vi "plot&save.vi"() -> ()   [LabVIEW 2019]
uses:
  <vilib>/Instr/_visa.llb/VISA Configure Serial Port (Instr).vi
panel:
  in  "Choose the data.txt file in the folder":path
  out "Muscle Activity":i32(graph)
  in  "?":bool
  in  "Conect your Arduino and choose the COM port":refnum<visa-resource-name>
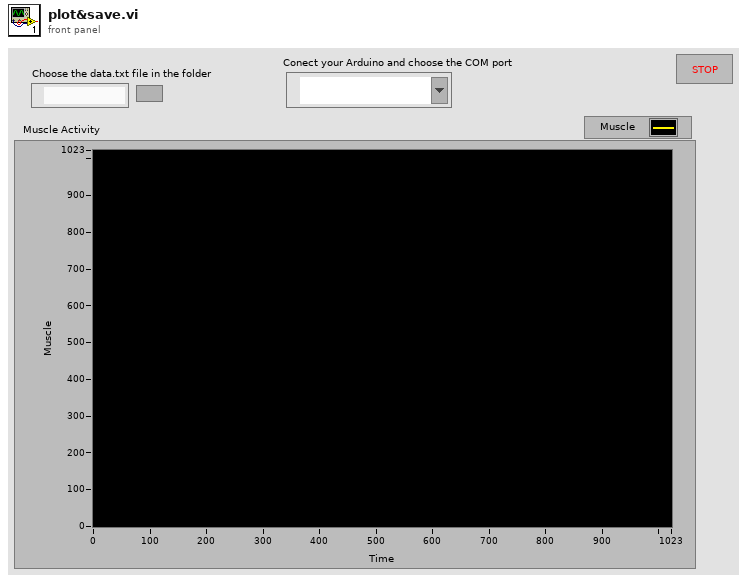
[diagram p1: front panel]
types:
  T1 = enum16{"open", "replace", "create", "open or create", "replace or create", "replace or create with confirmation"}
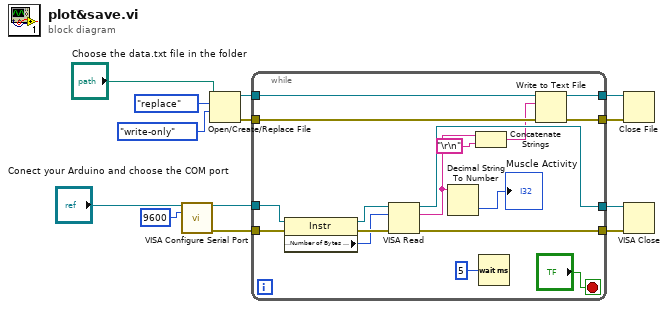
[diagram p0: block diagram]
diagram:
  n1 = call-poly "VISA Configure Serial Port"("VISA resource name"="Conect your Arduino and choose the COM port", "baud rate (9600)"=u32 9600) -> ("VISA resource name out"=w11:refnum<visa-resource-name>, "error out"=w10:errorcluster)  [unwired: 12 in]
  n2 = Open/Create/Replace File(file path (use dialog)="Choose the data.txt file in the folder", operation (0:open)=T1."replace", access (0:read/write)=enum16{"read/write", "read-only", "write-only"}."write-only") -> (refnum out=w7:refnum<file>, error out=w6:errorcluster)  [unwired: 3 in, 1 out]
  n3 = while {
    tunnel: w11 -> [w30]
    tunnel: w10 -> [w29]
    tunnel: [w28] -> w9
    tunnel: [w24] -> w8
    tunnel: w7 -> [w15]
    tunnel: w6 -> [w21]
    tunnel: [w20] -> w5
    tunnel: [w19] -> w4
    stop <- "?" stop-if-true
    n4 = property class="Instr"(reference=w30, error in=w29) -> (reference out=w27:refnum<visa-resource-name>, error out=w26:errorcluster, "Serial Settings:Number of Bytes at Serial Port"=w25:u32)
    n5 = VISA Read(VISA resource name=w27, byte count=w25, error in (no error)=w26) -> (VISA resource name out=w24:refnum<visa-resource-name>, read buffer=w18:string, error out=w28:errorcluster)  [unwired: 1 out]
    n6 = Decimal String To Number(string=w18) -> (number=→"Muscle Activity":i32)  [unwired: 2 in, 1 out]
    n7 = Concatenate Strings(w18, "\r\n") -> (w17:string)
    n8 = Wait (ms)(milliseconds to wait=u32 5) -> ()  [unwired: 1 out]
    n9 = Write to Text File(file (use dialog)=w15, text=w17, error in=w21) -> (refnum out=w20:refnum<file>, error out=w19:errorcluster)  [unwired: 1 in, 1 out]
  }
  n10 = Close File(refnum=w5, error in=w4) -> ()  [unwired: 2 out]
  n11 = VISA Close(VISA resource name=w8, error in (no error)=w9) -> ()  [unwired: 1 out]
